vi "Deconstruct LabVIEW Object.vi"(8 "error in (no error)":errorcluster, 10 "byte order (big-endian)":T2(ring)=enum."native, host order", 11 "flattened object":string) -> (0 "error out":errorcluster, 3 "LabVIEW Object Components":T1)   [LabVIEW 2016]
uses:
  LabVIEW Object Components.ctl
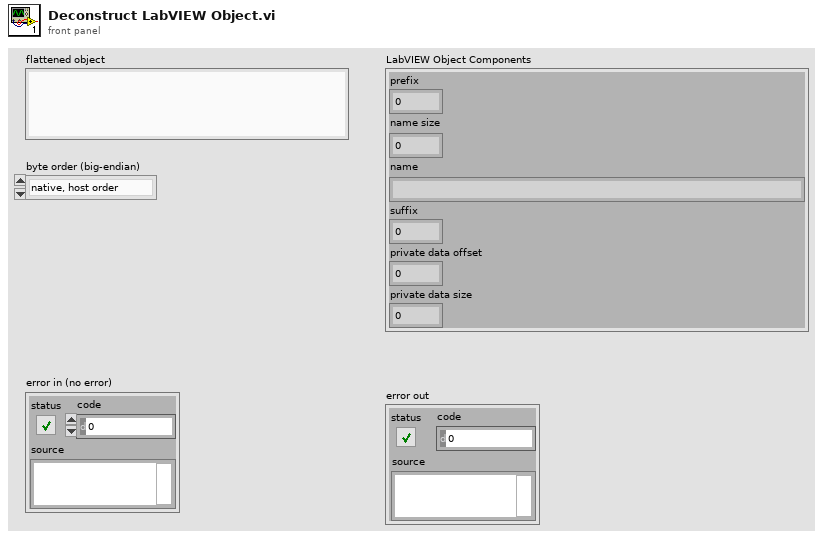
[diagram p1: front panel]
types:
  T1 = typedef "LabVIEW Object Components.ctl" = cluster{"prefix":i32, "name size":u8, "name":string, "suffix":u64, "private data offset":i32, "private data size":i32}
  T2 = enum16{"big-endian, network order", "native, host order", "little-endian"}
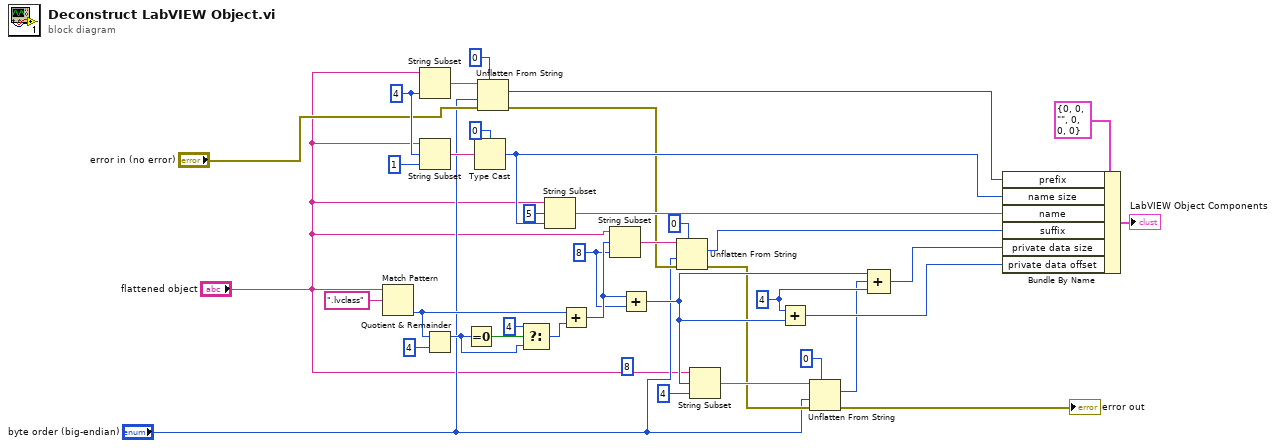
[diagram p0: block diagram]
diagram:
  w11 = 8 ("length (rest)")
  w22 = 4 ("length (rest)")
  w28 = 4 ("length (rest)")
  (unwired) 8 ("value")
  n1 = Match Pattern(string="flattened object", regular expression=".lvclass") -> (offset past match=w14:i32)  [unwired: 1 in, 3 out]
  n2 = String Subset(string="flattened object", length (rest)=w22) -> (substring=w25:string)  [unwired: 1 in]
  n3 = String Subset(string="flattened object", offset (0)=w22, length (rest)=1 ("length (rest)")) -> (substring=w20:string)
  n4 = Quotient & Remainder(x=w14, y=4) -> (x-y*floor(x/y)=w32:i32)  [unwired: 1 out]
  n5 = Equal To 0?(x=w32) -> (x = 0?=w33:bool)
  n6 = Type Cast(type=u8 0 ("prefix"), x=w20) -> (*(type *) &x=w15:u8)
  n7 = Unflatten From String(type=0 ("prefix"), binary string=w25, byte order (0:big-endian, network order)="byte order (big-endian)", error in (no error)="error in (no error)") -> (value=w23:i32, error out=w4:errorcluster)  [unwired: 1 in, 1 out]
  n8 = Select(t=4, s=w33, f=w32) -> (s? t:f=w13:i32)
  n9 = String Subset(string="flattened object", offset (0)=5, length (rest)=w15) -> (substring=w17:string)
  n10 = Add(x=w14, y=w13) -> (x+y=w12:i32)
  n11 = String Subset(string="flattened object", offset (0)=w12, length (rest)=w11) -> (substring=w7:string)
  n12 = Add(x=w12, y=w11) -> (x+y=w10:i32)
  n13 = Unflatten From String(type=u64 0 ("prefix"), binary string=w7, byte order (0:big-endian, network order)="byte order (big-endian)", error in (no error)=w4) -> (value=w6:u64, error out=w3:errorcluster)  [unwired: 1 in, 1 out]
  n14 = String Subset(string="flattened object", offset (0)=w10, length (rest)=4 ("length (rest)")) -> (substring=w35:string)
  n15 = Add(x=w28, y=w10) -> (x+y=w30:i32)
  n16 = Unflatten From String(type=0 ("length (rest)"), binary string=w35, byte order (0:big-endian, network order)="byte order (big-endian)", error in (no error)=w3) -> (value=w5:i32, error out=→"error out":errorcluster)  [unwired: 1 in, 1 out]
  n17 = Compound Arithmetic op=ADD(w10, w5, w28) -> ()  [unwired: 1 out]
  n18 = Bundle By Name(cluster=T1 {"prefix"=0, "name size"=0, "name"="", "suffix"=0, "private data offset"=0, "private data size"=0} ("LabVIEW Object Components"), "prefix"=w23, "name size"=w15, "name"=w17, "suffix"=w6, "private data size"=w5, "private data offset"=w30) -> (→"LabVIEW Object Components":T1)
